vi "Set Out.vi"(8 "error in (no error)":errorcluster, 10 "Output value":refnum<class "Output Value.lvclass">, 11 "Cryo-Con Driver in":refnum<class "Cryo-Con Driver.lvclass">) -> (0 "error out":errorcluster, 3 "Cryo-Con Driver out":refnum<class "Cryo-Con Driver.lvclass">)   [LabVIEW 2016, in "Cryo-Con Driver.lvclass"]
uses:
  Cryo-Con Driver.lvclass
  C:/github/NHMFL_Core/Libraries/Instruments/VISA Instrument/VISA Instrument.lvclass
  Utilities/Output Value/Output Value.lvclass
  C:/github/NHMFL_Core/Libraries/Instruments/Results/Acquired Result/Acquired Result.lvclass
  VISA Instrument/VISA Instrument.lvclass/VISA Instrument.ctl
  VISA Instrument/Read VISA resource.vi
  VISA Instrument/Write VISA resource.vi
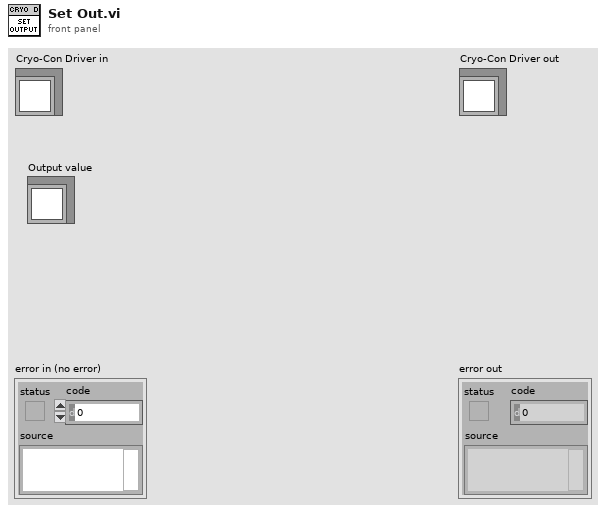
[diagram p1: front panel]
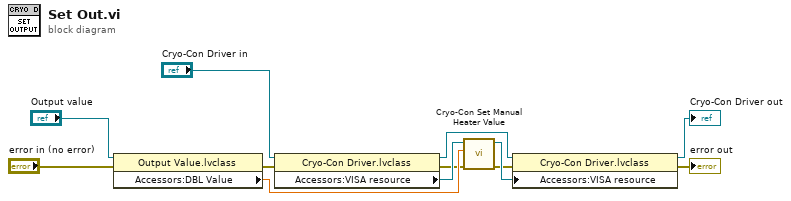
[diagram p0: block diagram]
diagram:
  n1 = property class="Output Value.lvclass"(reference="Output value", error in="error in (no error)") -> (error out=w5:errorcluster, "Accessors:DBL Value"=w6:dbl)  [unwired: 1 out]
  n2 = property class="Cryo-Con Driver.lvclass"(reference="Cryo-Con Driver in", error in=w5) -> (reference out=w9:refnum<class "Cryo-Con Driver.lvclass">, error out=w3:errorcluster, "Accessors:VISA resource"=w11:refnum<visa-resource-name>)
  n3 = call "Cryo-Con Set Manual Heater Value.vi"("error in (no error)"=w3, "Set heat %"=w6, "VISA Resource Name 2"=w11) -> ("error out"=w2:errorcluster, "VISA Resource Name Out"=w10:refnum<visa-resource-name>)  [unwired: 6 in, 1 out]
  n4 = property class="Cryo-Con Driver.lvclass"(reference=w9, error in=w2, "Accessors:VISA resource"=w10) -> (reference out=→"Cryo-Con Driver out":refnum<class "Cryo-Con Driver.lvclass">, error out=→"error out":errorcluster)
